vi "SVT Weighting Filter (octave) (1 Ch).vi"(0 "octave spectrum":T5 {"band power" format="%.2f"; "nominal frequencies [Hz]" format="%.2f"}, 5 "weighting":u16(ring) items=["Linear", "A-weighting", "B-weighting", "C-weighting"], 9 "octave info in":T1={"standard"=enum."ANSI S1.11", "bandwidth"=enum."1 octave", "low band"=0, "high band"=0, "weighting filter"=0, "dB reference"=0.0, "dB On"=FALSE, "unit label"="", "channel name"="", "description"="", "engineering units"=1, "custom label"="", "spectrum type"=enum."magnitude", "spectral density"=FALSE, "filters settled"=FALSE} {"engineering units" items=["custom..."=0, "V"=1, "A"=21, "C"=30, "pC"=31, "s"=32, "-"=29, "Pa"=2, "N"=20, "g"=3, "m/s^2"=4, "m/s"=5, "m"=6, "mm/s"=12, "mm"=13, "micron/s"=14, "micron"=15, "in/s^2"=7, "in/s"=8, "in"=9, "mil/s"=10, "mil"=11, "rad/s^2"=16, "rad/s"=17, "rad"=18, "deg/s^2"=26, "deg/s"=27, "deg"=28, "RPM"=22, "cycle/s^2"=23, "Hz"=24, "cycle"=25, "strain"=19]; "dB reference" format="%.2e"; "weighting filter" items=["Linear", "A-weighting", "B-weighting", "C-weighting", "ITU-R 468-4", "Dolby", "CCITT", "C-message", "Wb", "Wc", "Wd", "We", "Wf", "Wh", "Wj", "Wk", "Wm", "AES17 20 kHz lowpass", "AES17 40 kHz lowpass", "AES17 20 kHz highpass", "AES17 40 kHz highpass"]}, 11 "error in (no error)":errorcluster) -> (4 "weighted octave spectrum":T5 {"band power" format="%.2f"; "nominal frequencies [Hz]" format="%.2f"}, 6 "unit label":string, 8 "total band power":dbl format="%.2f", 10 "octave info out":T1={"standard"=enum."ANSI S1.11", "bandwidth"=enum."1 octave", "low band"=0, "high band"=0, "weighting filter"=0, "dB reference"=0.0, "dB On"=FALSE, "unit label"="", "channel name"="", "description"="", "engineering units"=1, "custom label"="", "spectrum type"=enum."magnitude", "spectral density"=FALSE, "filters settled"=FALSE} {"engineering units" items=["custom..."=0, "V"=1, "A"=21, "C"=30, "pC"=31, "s"=32, "-"=29, "Pa"=2, "N"=20, "g"=3, "m/s^2"=4, "m/s"=5, "m"=6, "mm/s"=12, "mm"=13, "micron/s"=14, "micron"=15, "in/s^2"=7, "in/s"=8, "in"=9, "mil/s"=10, "mil"=11, "rad/s^2"=16, "rad/s"=17, "rad"=18, "deg/s^2"=26, "deg/s"=27, "deg"=28, "RPM"=22, "cycle/s^2"=23, "Hz"=24, "cycle"=25, "strain"=19]; "dB reference" format="%.2e"; "weighting filter" items=["Linear", "A-weighting", "B-weighting", "C-weighting", "ITU-R 468-4", "Dolby", "CCITT", "C-message", "Wb", "Wc", "Wd", "We", "Wf", "Wh", "Wj", "Wk", "Wm", "AES17 20 kHz lowpass", "AES17 40 kHz lowpass", "AES17 20 kHz highpass", "AES17 40 kHz highpass"]}, 15 "error out":errorcluster)   [LabVIEW 2017, in "SoundVib_Octave_2014 standard.lvlib"]
doc: "Applies the selected weighting to a previously computed <B>octave spectrum</B> or <B>octave spectra</B>. This VI weights each spectral bin according to the attenuation of the specified filter at the bin center frequency. You can use this VI in a loop to process multiple blocks. Wire data to the <B>octave spectrum</B> input to determine the polymorphic instance to use or manually select the instance."
uses:
  <vilib>/addons/Sound and Vibration/svt_Octave/SoundVib_Octave_2014 standard.lvlib
  <vilib>/addons/_NISVFA/_Shared subVIs/Controls/svc_Octave Info.ctl
  <vilib>/addons/_NISVFA/_Shared subVIs/Controls/svc_Octave Standard.ctl
  <vilib>/addons/_NISVFA/_Shared subVIs/Controls/svc_Weighting Filter Text Ring.ctl
  <vilib>/addons/_NISVFA/_Shared subVIs/Controls/svc_Engineering Units Text Ring.ctl
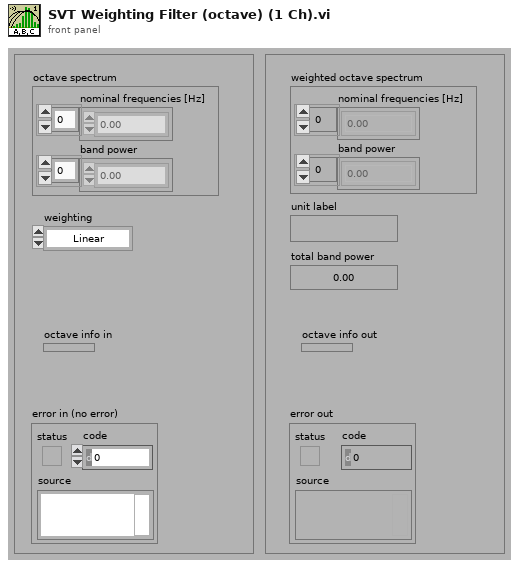
[diagram p1: front panel]
types:
  T1 = typedef "svc_Octave Info.ctl" = cluster{"standard":T2, "bandwidth":enum16{"1 octave", "1/3 octave", "1/6 octave", "1/12 octave", "1/24 octave"}, "low band":i32, "high band":i32, "weighting filter":T3, "dB reference":dbl, "dB On":bool, "unit label":string, "channel name":string, "description":string, "engineering units":T4, "custom label":string, "spectrum type":enum16{"power", "magnitude"}, "spectral density":bool, "filters settled":bool}
  T2 = typedef "svc_Octave Standard.ctl" = enum16{"ANSI S1.11", "IEC 61260"}
  T3 = typedef "svc_Weighting Filter Text Ring.ctl" = u16
  T4 = typedef "svc_Engineering Units Text Ring.ctl" = u16
  T5 = cluster{"nominal frequencies [Hz]":dbl[], "band power":dbl[]}
  T6 = cluster{"nominal frequencies [Hz]":dbl[], "band power [dB EU]":dbl[]}
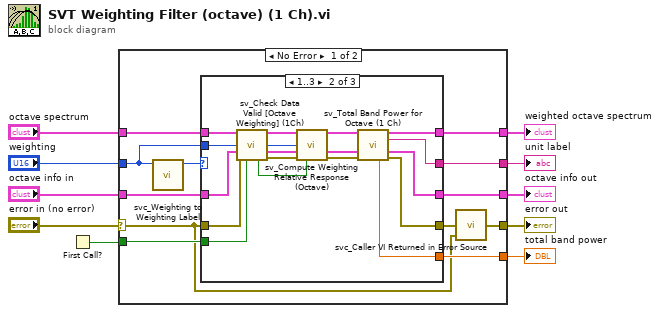
[diagram p0: block diagram]
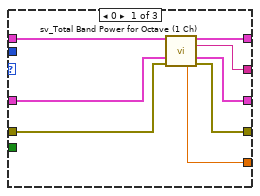
[diagram p2: hidden frame]
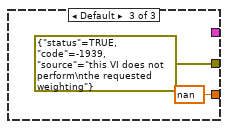
[diagram p3: hidden frame]
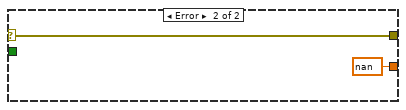
[diagram p4: hidden frame]
diagram:
  n1 = First Call?() -> (First Call?: T/F=w2:bool)
  n2 = case shown="No Error" "error in (no error)" {
    selector: "error in (no error)" -> [w11 w52]
    tunnel: [w21 w52] -> w9
    tunnel: "weighting" -> [w14 _]
    tunnel: [w22 _] -> w6
    tunnel: "octave spectrum" -> [w18 _]
    tunnel: [w19 _] -> w7
    tunnel: "octave info in" -> [w16 _]
    tunnel: [w20 _] -> w3
    tunnel: w2 -> [w17 _]
    tunnel: [w12 nan ("total band power [dB EU]")] -> w1
    frame No Error {
      n3 = call <vilib>:"svc_Weighting to Weighting Label.vi"("weighting filter"=w14) -> ("weighting enum"=w13:T3)  [unwired: 9 in, 1 out]
      n4 = case shown="1..3" w13 {
        tunnel: [w29 w37 _] -> w22
        tunnel: [w25 w33 _] -> w20
        tunnel: [w26 w32 _] -> w19
        tunnel: w18 -> [w30 w48 _]
        tunnel: w11 -> [w27 w46 _]
        tunnel: w17 -> [_ w45 _]
        tunnel: w14 -> [_ w44 _]
        tunnel: w16 -> [w28 w43 _]
        tunnel: [w24 w34 errorcluster {"status"=TRUE, "code"=-1939, "source"="this VI does not perform\nthe requested weighting"} ("error out")] -> w15
        tunnel: [w23 w31 nan ("total band power [dB EU]")] -> w12
        frame 0 {
          n5 = call <vilib>:"sv_Total Band Power for Octave (1 Ch).vi"("octave spectrum"=w30, "octave info"=w28, "error in (no error)"=w27) -> ("dup octave spectrum"=w29:T6, "unit label"=w26:string, "dup octave info"=w25:T1, "total band power [dB EU]"=w23:dbl, "error out"=w24:errorcluster)  [unwired: 8 in]
        }
        frame 1..3 {
          n6 = call <vilib>:"sv_Check Data Valid [Octave Weighting] (1Ch).vi"("octave spectrum"=w48, "weighting filter"=w44, "octave info in"=w43, "error in (no error)"=w46, "reset in"=w45) -> ("dup octave spectrum"=w47:T6, "dup weighting filter"=w40:u16, "octave info in"=w42:T1, "reset out"=w41:bool, "error out"=w39:errorcluster)  [unwired: 6 in]
          n7 = call <vilib>:"sv_Compute Weighting Relative Response (Octave).vi"("octave spectrum"=w47, "weighting filter"=w40, "octave info in"=w42, "error in (no error)"=w39, "reset"=w41) -> ("weighted octave spectrum"=w38:T6, "octave info out"=w36:T1, "error out"=w35:errorcluster)  [unwired: 8 in]
          n8 = call <vilib>:"sv_Total Band Power for Octave (1 Ch).vi"("octave spectrum"=w38, "octave info"=w36, "error in (no error)"=w35) -> ("dup octave spectrum"=w37:T6, "unit label"=w32:string, "dup octave info"=w33:T1, "total band power [dB EU]"=w31:dbl, "error out"=w34:errorcluster)  [unwired: 8 in]
        }
        frame Default {
        }
      }
      n9 = call <vilib>:"svc_Caller VI Returned in Error Source.vi"("warning input to caller"=w11, "error in (no error)"=w15) -> ("error out"=w21:errorcluster)  [unwired: 3 in]
    }
    frame Error {
    }
  }
  "error out" <- w9
  "weighted octave spectrum" <- w6
  "unit label" <- w7
  "octave info out" <- w3
  "total band power" <- w1
